vi "Termo_1.5__.vi"() -> ()   [LabVIEW 2015]
doc: "Программа мониторинга температуры и вакуума"
uses:
  tango_vi.llb/avToDoubleScalar.vi
  tango_vi.llb/tango.lvlib
panel:
  out "T1":dbl format="%.2f"
  out "C2":string
  out "C1":string
  out "Т3":dbl format="%.2f"
  out "Т5":dbl format="%.2f"
  out "Т8":dbl format="%.2f"
  out "Т6":dbl format="%.2f"
  out "T14":dbl format="%.2f"
  out "T13":dbl format="%.2f"
  out "Т9":dbl format="%.2f"
  out "Т7":dbl format="%.2f"
  out "PKT2 state":u32(colorbox) caption="ON"
  out "PKT1 state":u32(colorbox) caption="ON"
  out "device name 2":string="kriontube/termo/pkt2"
  out "attribute names 3":string[](array[string])=["R1", "R2", "R3", "R4", "R5", "R6", "R7", "R8"]
  out "Tango device name":string="kriontube/termo/pkt1"
  out "attribute names 2":string[](array[string])=["T1", "T2", "T3", "T4", "T5", "T6", "T7", "T8"]
  out "attribute names":string[](array[string])=["s1_status_byte", "sensor1_P", "sensor2_P", "s2_status_byte"]
  out "Tango device name":string="kriontube/vacuum/tpg361"
  out "Последнее обновление :":string
  out "S 2":string
  out "S 1":string
  out "R13":dbl format="%.2f"
  in  "stop":bool
  out "R9":dbl format="%.2f"
  out "R10":dbl format="%.2f"
  out "R11":dbl format="%.2f"
  out "R12":dbl format="%.2f"
  out "R14":dbl format="%.2f"
  out "R7":dbl format="%.2f"
  out "R5":dbl format="%.2f"
  out "R8":dbl format="%.2f"
  out "R6":dbl format="%.2f"
  out "R3":dbl format="%.2f"
  out "R1":dbl format="%.2f"
  out "R4":dbl format="%.2f"
  out "R2":dbl format="%.2f"
  out "R16":dbl format="%.2f"
  out "R15":dbl format="%.2f"
  out "T12":dbl format="%.2f"
  out "T10":dbl format="%.2f"
  out "T11":dbl format="%.2f"
  out "T4":dbl format="%.2f"
  out "T2":dbl format="%.2f"
  out "TPG 361 state":u32(colorbox) caption="UNKNOWN"
  out "T15":dbl format="%.2f"
  out "T16":dbl format="%.2f"
  # "КРИОН-Т"
  # "4 K"
  # "40 K"
  # "P"
  # "[ mBar ]"
  # "R [Ом]"
  # "R1"
  # "R2"
  # "R3"
  # "R4"
  # "R5"
  # "R6"
  # "R7"
  # "R9"
  # "R8"
  # "R10"
  # "R11"
  # "T1"
  # "R12"
  # "R13"
  # "R14"
  # "Вакуум"
  # "Термометрия \nПКТ8-1 , ПКТ8-2"
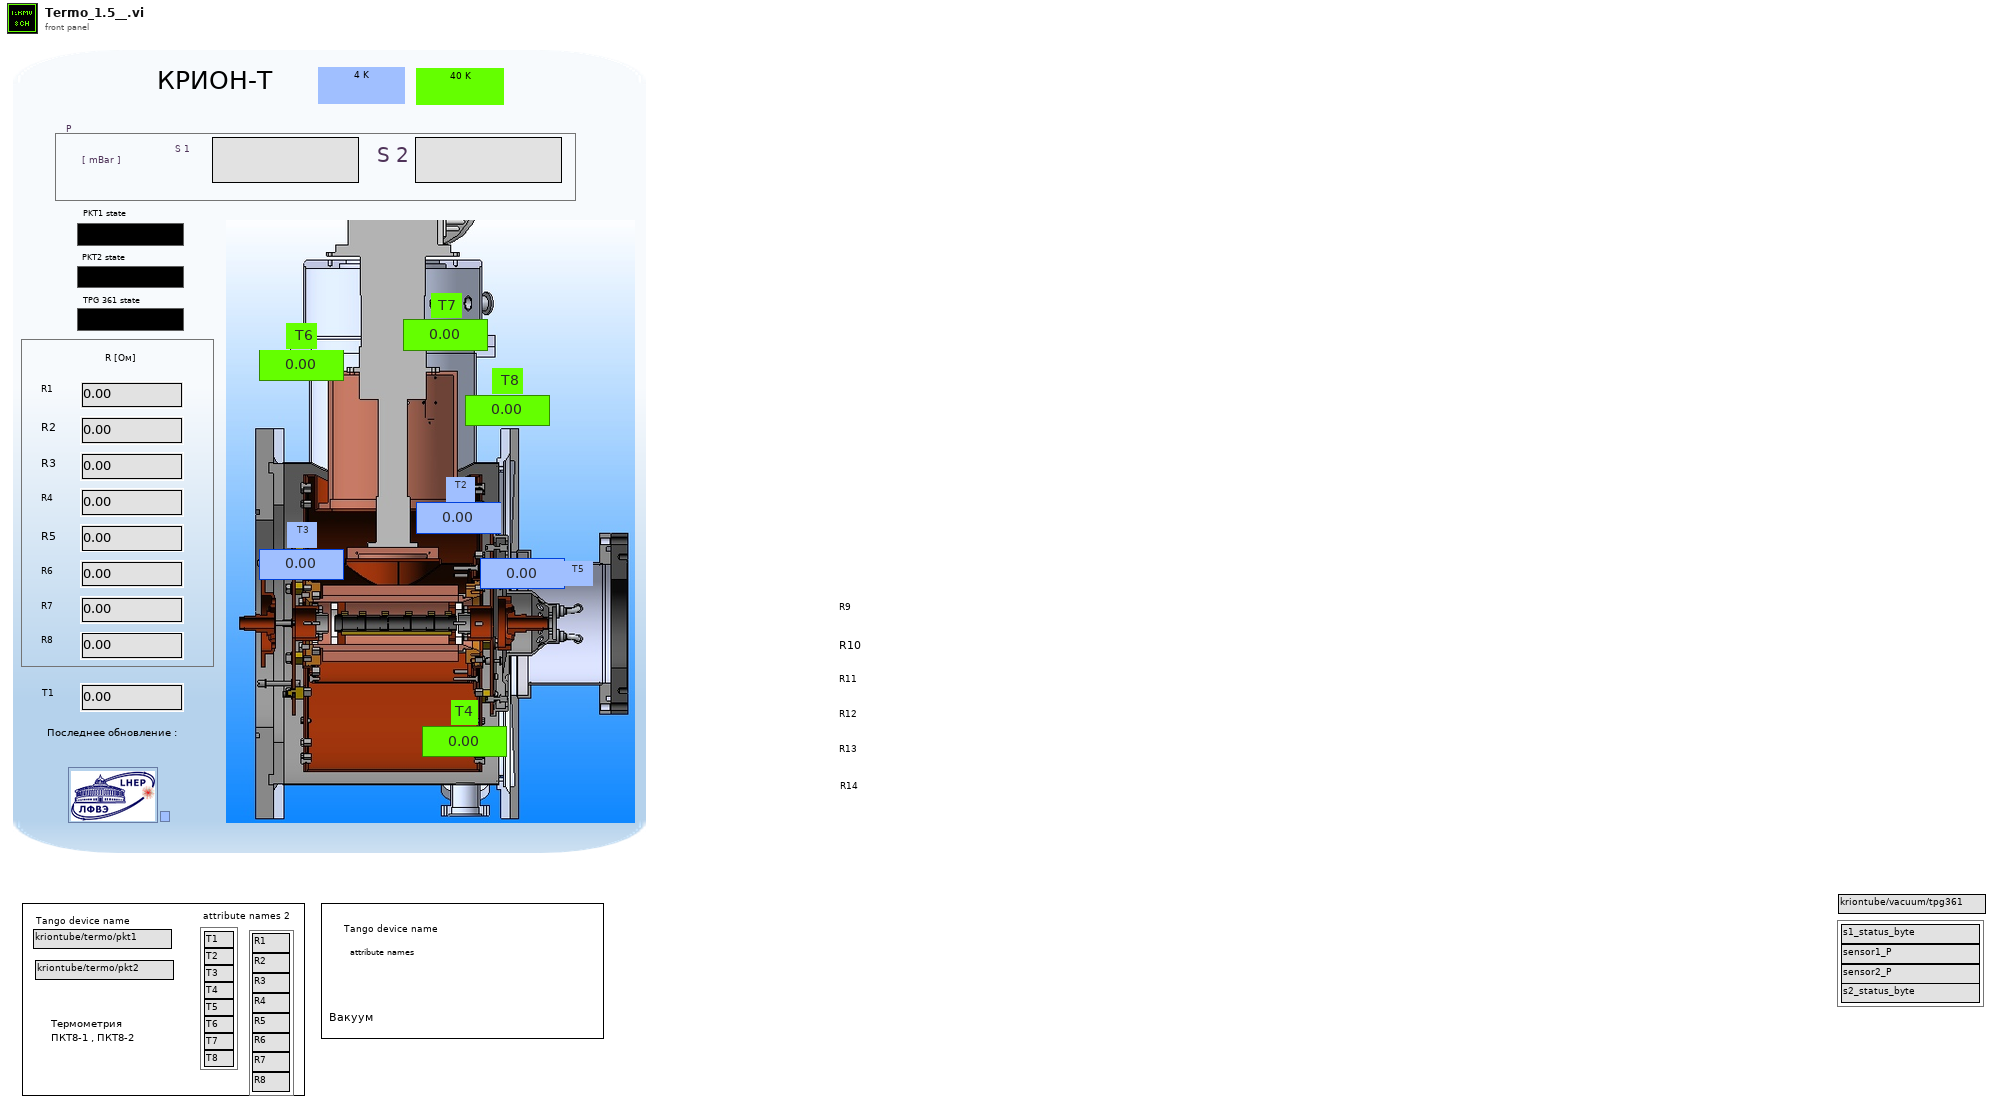
[diagram p1: front panel]
types:
  T1 = cluster{"device name":string, "attribute name":string, "quality value":i16, "quality string":string, "timestamp":dbl, "dim. x":i32, "dim. y":i32, "value":u8[], "error code":i32, "error stack":string[], "data type":u16}[]
  T2 = cluster{"device name":string, "attribute name":string, "quality value":i16, "quality string":string, "timestamp":dbl, "dim. x":i32, "dim. y":i32, "value":u8[], "error code":i32, "error stack":string[], "data type":u16}
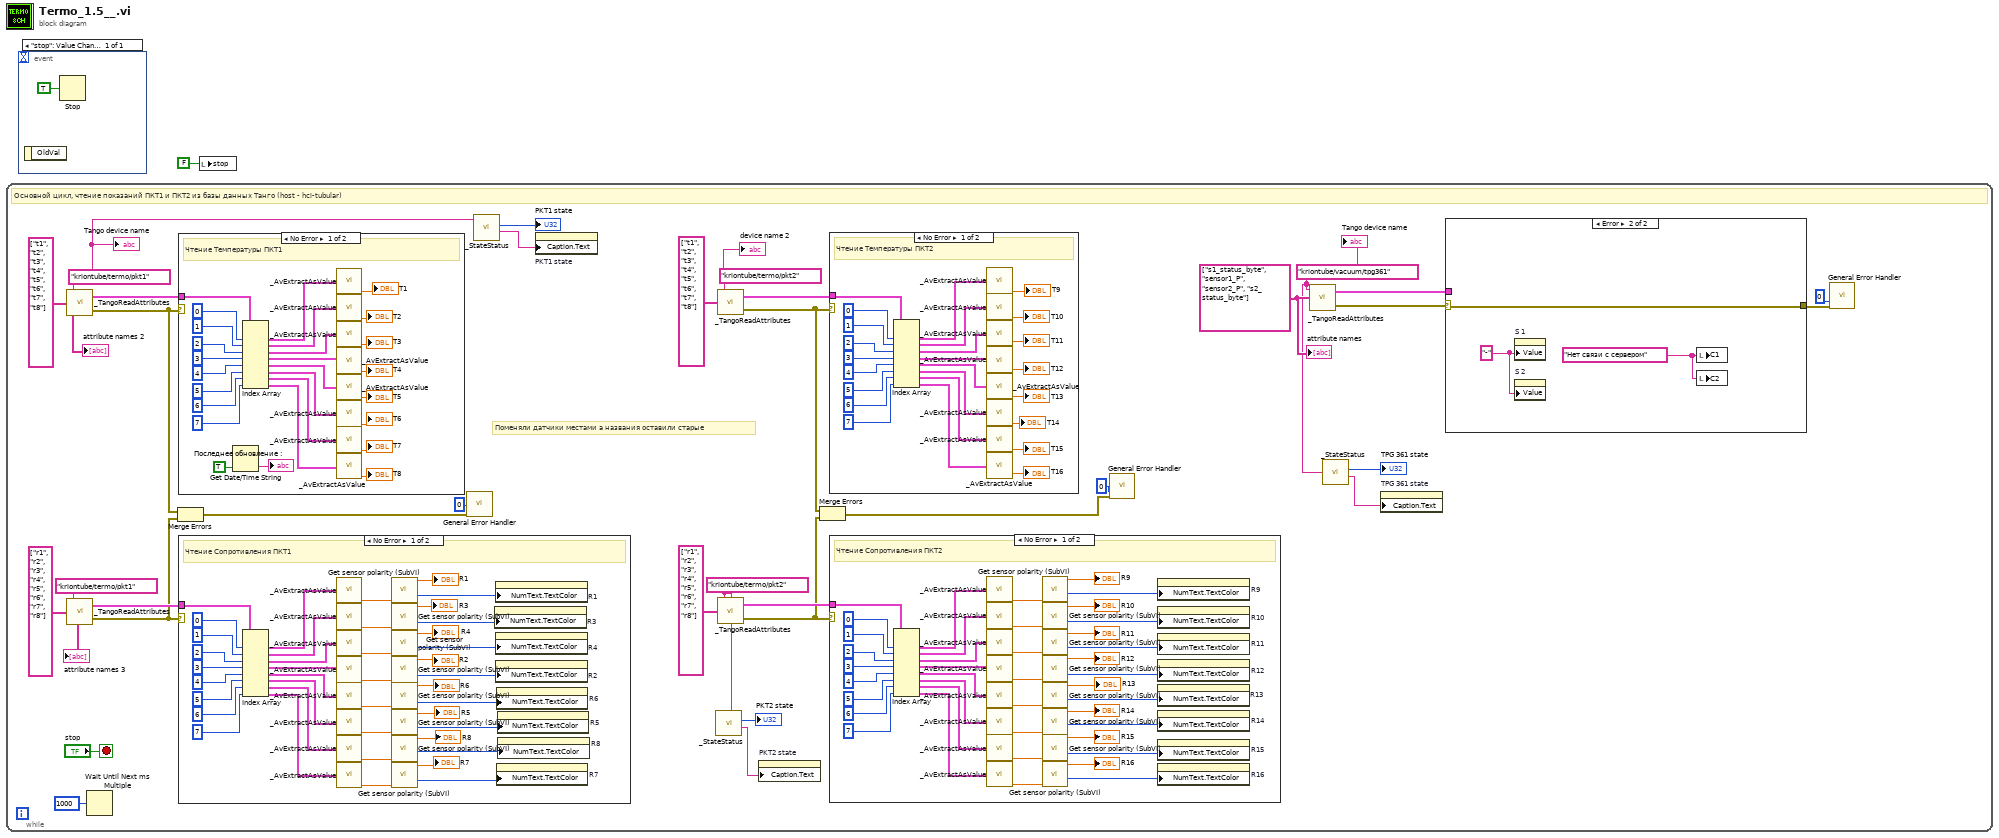
[diagram p0: block diagram]
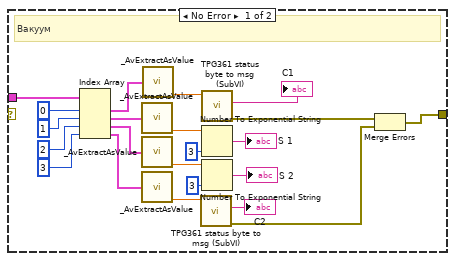
[diagram p2: hidden frame]
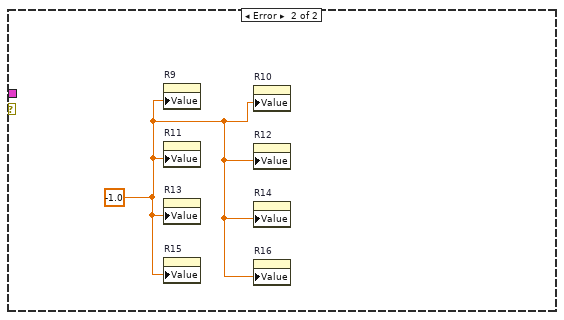
[diagram p3: hidden frame]
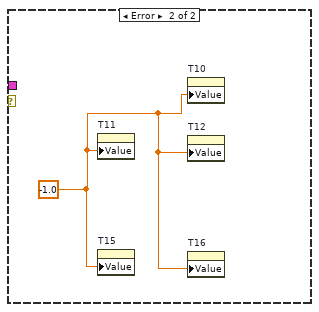
[diagram p4: hidden frame]
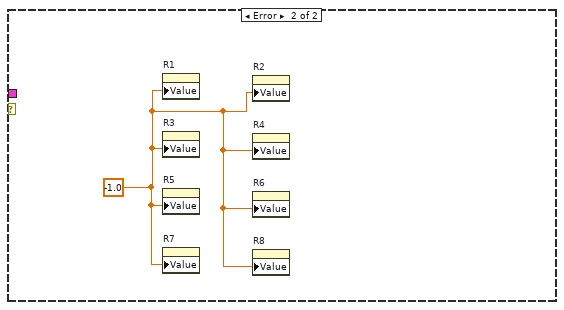
[diagram p5: hidden frame]
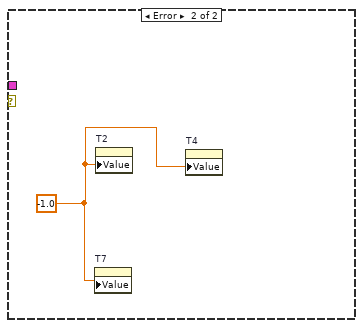
[diagram p6: hidden frame]
diagram:
  n1 = while {
    stop <- "stop" stop-if-true
    w14 = string[] ["s1_status_byte", "sensor1_P", "sensor2_P", "s2_status_byte"] ("attribute names")
    w2 = "kriontube/vacuum/tpg361" ("device name")
    w7 = "kriontube/termo/pkt2" ("device name")
    w26 = "kriontube/termo/pkt2" ("device name")
    w30 = string[] ["r1", "r2", "r3", "r4", "r5", "r6", "r7", "r8"] ("attribute names")
    w11 = "kriontube/termo/pkt1" ("device name")
    w31 = string[] ["t1", "t2", "t3", "t4", "t5", "t6", "t7", "t8"] ("attribute names")
    # "Поменяли датчики местами а названия оставили старые"
    # "Основной цикл, чтение показаний ПКТ1 и ПКТ2 из базы данных Танго (host - hci-tubular)"
    n2 = call "_TangoReadAttributes.vi"("attribute names"=w31, "device name"=w11) -> ("error out"=w23:errorcluster, "attribute values"=w32:T1)  [unwired: 1 in]
    n3 = call "_TangoReadAttributes.vi"("attribute names"=w30, "device name"="kriontube/termo/pkt1") -> ("error out"=w22:errorcluster, "attribute values"=w29:T1)  [unwired: 1 in]
    n4 = Wait Until Next ms Multiple(millisecond multiple=u32 1000) -> ()  [unwired: 1 out]
    n5 = Merge Errors(w23, w22) -> (w21:errorcluster)
    n6 = case shown="No Error" w23 {
      tunnel: w32 -> [w196 _]
      frame No Error {
        # "Чтение Температуры ПКТ1"
        n7 = Get Date/Time String(want seconds? (F)=TRUE) -> (time string=→"Последнее обновление :":string)  [unwired: 2 in, 1 out]
        n8 = Index Array(array=w196, index #1=0 ("indice"), index #2=1 ("index"), index #3=2 ("indice"), index #4=3 ("index"), index #5=4 ("index"), index #6=5 ("indice"), index #7=6 ("index"), index #8=7 ("indice")) -> (element #1=w195:T2, element #2=w190:T2, element #3=w189:T2, element #4=w188:T2, element #5=w187:T2, element #6=w183:T2, element #7=w182:T2, element #8=w181:T2)
        n9 = call-poly "_AvExtractAsValue.vi"("attribute value"=w195) -> ("value"=→"T1":dbl)  [unwired: 4 out]
        n10 = call-poly "_AvExtractAsValue.vi"("attribute value"=w190) -> ("value"=→"T2":dbl)  [unwired: 4 out]
        n11 = call-poly "_AvExtractAsValue.vi"("attribute value"=w189) -> ("value"=→"Т3":dbl)  [unwired: 4 out]
        n12 = call-poly "_AvExtractAsValue.vi"("attribute value"=w188) -> ("value"=→"T4":dbl)  [unwired: 4 out]
        n13 = call-poly "_AvExtractAsValue.vi"("attribute value"=w187) -> ("value"=→"Т5":dbl)  [unwired: 4 out]
        n14 = call-poly "_AvExtractAsValue.vi"("attribute value"=w183) -> ("value"=→"Т6":dbl)  [unwired: 4 out]
        n15 = call-poly "_AvExtractAsValue.vi"("attribute value"=w182) -> ("value"=→"Т7":dbl)  [unwired: 4 out]
        n16 = call-poly "_AvExtractAsValue.vi"("attribute value"=w181) -> ("value"=→"Т8":dbl)  [unwired: 4 out]
      }
      frame Error {
        w198 = -1.0 ("millisecond multiple")
        n17 = property on="Т7" class="DigNum (strict)"("Value"=w198) -> ()  [unwired: 2 in, 2 out]
        n18 = property on="T2" class="DigNum (strict)"("Value"=w198) -> ()  [unwired: 2 in, 2 out]
        n19 = property on="T4" class="DigNum (strict)"("Value"=w198) -> ()  [unwired: 2 in, 2 out]
      }
    }
    n20 = case shown="No Error" w22 {
      tunnel: w29 -> [w168 _]
      frame No Error {
        # "Чтение Сопротивления ПКТ1"
        n21 = Index Array(array=w168, index #1=0 ("indice"), index #2=1 ("index"), index #3=2 ("indice"), index #4=3 ("index"), index #5=4 ("index"), index #6=5 ("indice"), index #7=6 ("index"), index #8=7 ("indice")) -> (element #1=w167:T2, element #2=w162:T2, element #3=w161:T2, element #4=w160:T2, element #5=w159:T2, element #6=w155:T2, element #7=w154:T2, element #8=w153:T2)
        n22 = call-poly "_AvExtractAsValue.vi"("attribute value"=w167) -> ("value"=w152:dbl)  [unwired: 4 out]
        n23 = call-poly "_AvExtractAsValue.vi"("attribute value"=w162) -> ("value"=w151:dbl)  [unwired: 4 out]
        n24 = call-poly "_AvExtractAsValue.vi"("attribute value"=w161) -> ("value"=w150:dbl)  [unwired: 4 out]
        n25 = call-poly "_AvExtractAsValue.vi"("attribute value"=w160) -> ("value"=w149:dbl)  [unwired: 4 out]
        n26 = call-poly "_AvExtractAsValue.vi"("attribute value"=w159) -> ("value"=w148:dbl)  [unwired: 4 out]
        n27 = call-poly "_AvExtractAsValue.vi"("attribute value"=w155) -> ("value"=w147:dbl)  [unwired: 4 out]
        n28 = call-poly "_AvExtractAsValue.vi"("attribute value"=w154) -> ("value"=w146:dbl)  [unwired: 4 out]
        n29 = call-poly "_AvExtractAsValue.vi"("attribute value"=w153) -> ("value"=w145:dbl)  [unwired: 4 out]
        n30 = call "Get sensor polarity (SubVI).vi"("R вх"=w152) -> ("R по модулю"=→"R1":dbl, "Цвет полярности вкл. R"=w143:u32)  [unwired: 13 in]
        n31 = call "Get sensor polarity (SubVI).vi"("R вх"=w151) -> ("R по модулю"=→"R3":dbl, "Цвет полярности вкл. R"=w141:u32)  [unwired: 13 in]
        n32 = call "Get sensor polarity (SubVI).vi"("R вх"=w150) -> ("R по модулю"=→"R4":dbl, "Цвет полярности вкл. R"=w139:u32)  [unwired: 13 in]
        n33 = call "Get sensor polarity (SubVI).vi"("R вх"=w149) -> ("R по модулю"=→"R2":dbl, "Цвет полярности вкл. R"=w137:u32)  [unwired: 13 in]
        n34 = call "Get sensor polarity (SubVI).vi"("R вх"=w148) -> ("R по модулю"=→"R6":dbl, "Цвет полярности вкл. R"=w135:u32)  [unwired: 13 in]
        n35 = call "Get sensor polarity (SubVI).vi"("R вх"=w147) -> ("R по модулю"=→"R5":dbl, "Цвет полярности вкл. R"=w133:u32)  [unwired: 13 in]
        n36 = call "Get sensor polarity (SubVI).vi"("R вх"=w146) -> ("R по модулю"=→"R8":dbl, "Цвет полярности вкл. R"=w131:u32)  [unwired: 13 in]
        n37 = call "Get sensor polarity (SubVI).vi"("R вх"=w145) -> ("R по модулю"=→"R7":dbl, "Цвет полярности вкл. R"=w129:u32)  [unwired: 13 in]
        n38 = property on="R3" class="DigNum (strict)"("NumText.TextColor"=w141) -> ()  [unwired: 2 in, 2 out]
        n39 = property on="R1" class="DigNum (strict)"("NumText.TextColor"=w143) -> ()  [unwired: 2 in, 2 out]
        n40 = property on="R4" class="DigNum (strict)"("NumText.TextColor"=w139) -> ()  [unwired: 2 in, 2 out]
        n41 = property on="R2" class="DigNum (strict)"("NumText.TextColor"=w137) -> ()  [unwired: 2 in, 2 out]
        n42 = property on="R6" class="DigNum (strict)"("NumText.TextColor"=w135) -> ()  [unwired: 2 in, 2 out]
        n43 = property on="R7" class="DigNum (strict)"("NumText.TextColor"=w129) -> ()  [unwired: 2 in, 2 out]
        n44 = property on="R5" class="DigNum (strict)"("NumText.TextColor"=w133) -> ()  [unwired: 2 in, 2 out]
        n45 = property on="R8" class="DigNum (strict)"("NumText.TextColor"=w131) -> ()  [unwired: 2 in, 2 out]
      }
      frame Error {
        w170 = -1.0 ("millisecond multiple")
        n46 = property on="R1" class="DigNum (strict)"("Value"=w170) -> ()  [unwired: 2 in, 2 out]
        n47 = property on="R3" class="DigNum (strict)"("Value"=w170) -> ()  [unwired: 2 in, 2 out]
        n48 = property on="R5" class="DigNum (strict)"("Value"=w170) -> ()  [unwired: 2 in, 2 out]
        n49 = property on="R7" class="DigNum (strict)"("Value"=w170) -> ()  [unwired: 2 in, 2 out]
        n50 = property on="R2" class="DigNum (strict)"("Value"=w170) -> ()  [unwired: 2 in, 2 out]
        n51 = property on="R4" class="DigNum (strict)"("Value"=w170) -> ()  [unwired: 2 in, 2 out]
        n52 = property on="R6" class="DigNum (strict)"("Value"=w170) -> ()  [unwired: 2 in, 2 out]
        n53 = property on="R8" class="DigNum (strict)"("Value"=w170) -> ()  [unwired: 2 in, 2 out]
      }
    }
    n54 = call <vilib>:"General Error Handler.vi"("type of dialog (OK msg:1)"=u32 0 ("milliseconds to wait"), "error in (no error)"=w21) -> ()  [unwired: 1 in, 13 out]
    n55 = call "_StateStatus.vi"("Device Name"=w11) -> ("State Color"=→"PKT1 state":u32, "State String"=w6:string)  [unwired: 4 out]
    n56 = property on="PKT1 state" class="ColBox"("Caption.Text"=w6) -> ()  [unwired: 2 in, 2 out]
    n57 = call "_StateStatus.vi"("Device Name"=w7) -> ("State Color"=→"PKT2 state":u32, "State String"=w5:string)  [unwired: 4 out]
    n58 = call "_TangoReadAttributes.vi"("attribute names"=string[] ["t1", "t2", "t3", "t4", "t5", "t6", "t7", "t8"], "device name"=w26) -> ("error out"=w19:errorcluster, "attribute values"=w24:T1)  [unwired: 1 in]
    n59 = call "_TangoReadAttributes.vi"("attribute names"=string[] ["r1", "r2", "r3", "r4", "r5", "r6", "r7", "r8"], "device name"=w7) -> ("error out"=w18:errorcluster, "attribute values"=w28:T1)  [unwired: 1 in]
    n60 = property on="PKT2 state" class="ColBox"("Caption.Text"=w5) -> ()  [unwired: 2 in, 2 out]
    n61 = Merge Errors(w19, w18) -> (w17:errorcluster)
    n62 = case shown="No Error" w19 {
      tunnel: w24 -> [w126 _]
      frame No Error {
        # "Чтение Температуры ПКТ2"
        n63 = Index Array(array=w126, index #1=0 ("indice"), index #2=1 ("index"), index #3=2 ("indice"), index #4=3 ("index"), index #5=4 ("index"), index #6=5 ("indice"), index #7=6 ("index"), index #8=7 ("indice")) -> (element #1=w125:T2, element #2=w120:T2, element #3=w119:T2, element #4=w118:T2, element #5=w117:T2, element #6=w113:T2, element #7=w112:T2, element #8=w111:T2)
        n64 = call-poly "_AvExtractAsValue.vi"("attribute value"=w125) -> ("value"=→"Т9":dbl)  [unwired: 4 out]
        n65 = call-poly "_AvExtractAsValue.vi"("attribute value"=w120) -> ("value"=→"T10":dbl)  [unwired: 4 out]
        n66 = call-poly "_AvExtractAsValue.vi"("attribute value"=w119) -> ("value"=→"T11":dbl)  [unwired: 4 out]
        n67 = call-poly "_AvExtractAsValue.vi"("attribute value"=w118) -> ("value"=→"T12":dbl)  [unwired: 4 out]
        n68 = call-poly "_AvExtractAsValue.vi"("attribute value"=w117) -> ("value"=→"T13":dbl)  [unwired: 4 out]
        n69 = call-poly "_AvExtractAsValue.vi"("attribute value"=w113) -> ("value"=→"T14":dbl)  [unwired: 4 out]
        n70 = call-poly "_AvExtractAsValue.vi"("attribute value"=w112) -> ("value"=→"T15":dbl)  [unwired: 4 out]
        n71 = call-poly "_AvExtractAsValue.vi"("attribute value"=w111) -> ("value"=→"T16":dbl)  [unwired: 4 out]
      }
      frame Error {
        w128 = -1.0 ("millisecond multiple")
        n72 = property on="T11" class="DigNum (strict)"("Value"=w128) -> ()  [unwired: 2 in, 2 out]
        n73 = property on="T15" class="DigNum (strict)"("Value"=w128) -> ()  [unwired: 2 in, 2 out]
        n74 = property on="T10" class="DigNum (strict)"("Value"=w128) -> ()  [unwired: 2 in, 2 out]
        n75 = property on="T12" class="DigNum (strict)"("Value"=w128) -> ()  [unwired: 2 in, 2 out]
        n76 = property on="T16" class="DigNum (strict)"("Value"=w128) -> ()  [unwired: 2 in, 2 out]
      }
    }
    n77 = case shown="No Error" w18 {
      tunnel: w28 -> [w100 _]
      frame No Error {
        # "Чтение Сопротивления ПКТ2"
        n78 = Index Array(array=w100, index #1=0 ("indice"), index #2=1 ("index"), index #3=2 ("indice"), index #4=3 ("index"), index #5=4 ("index"), index #6=5 ("indice"), index #7=6 ("index"), index #8=7 ("indice")) -> (element #1=w99:T2, element #2=w94:T2, element #3=w93:T2, element #4=w92:T2, element #5=w91:T2, element #6=w87:T2, element #7=w86:T2, element #8=w85:T2)
        n79 = call-poly "_AvExtractAsValue.vi"("attribute value"=w99) -> ("value"=w84:dbl)  [unwired: 4 out]
        n80 = call-poly "_AvExtractAsValue.vi"("attribute value"=w94) -> ("value"=w83:dbl)  [unwired: 4 out]
        n81 = call-poly "_AvExtractAsValue.vi"("attribute value"=w93) -> ("value"=w82:dbl)  [unwired: 4 out]
        n82 = call-poly "_AvExtractAsValue.vi"("attribute value"=w92) -> ("value"=w81:dbl)  [unwired: 4 out]
        n83 = call-poly "_AvExtractAsValue.vi"("attribute value"=w91) -> ("value"=w63:dbl)  [unwired: 4 out]
        n84 = call-poly "_AvExtractAsValue.vi"("attribute value"=w87) -> ("value"=w80:dbl)  [unwired: 4 out]
        n85 = call-poly "_AvExtractAsValue.vi"("attribute value"=w86) -> ("value"=w79:dbl)  [unwired: 4 out]
        n86 = call-poly "_AvExtractAsValue.vi"("attribute value"=w85) -> ("value"=w78:dbl)  [unwired: 4 out]
        n87 = call "Get sensor polarity (SubVI).vi"("R вх"=w84) -> ("R по модулю"=→"R9":dbl, "Цвет полярности вкл. R"=w70:u32)  [unwired: 13 in]
        n88 = call "Get sensor polarity (SubVI).vi"("R вх"=w83) -> ("R по модулю"=→"R10":dbl, "Цвет полярности вкл. R"=w69:u32)  [unwired: 13 in]
        n89 = call "Get sensor polarity (SubVI).vi"("R вх"=w82) -> ("R по модулю"=→"R11":dbl, "Цвет полярности вкл. R"=w68:u32)  [unwired: 13 in]
        n90 = call "Get sensor polarity (SubVI).vi"("R вх"=w81) -> ("R по модулю"=→"R12":dbl, "Цвет полярности вкл. R"=w67:u32)  [unwired: 13 in]
        n91 = call "Get sensor polarity (SubVI).vi"("R вх"=w63) -> ("R по модулю"=→"R13":dbl, "Цвет полярности вкл. R"=w61:u32)  [unwired: 13 in]
        n92 = call "Get sensor polarity (SubVI).vi"("R вх"=w80) -> ("R по модулю"=→"R14":dbl, "Цвет полярности вкл. R"=w66:u32)  [unwired: 13 in]
        n93 = call "Get sensor polarity (SubVI).vi"("R вх"=w79) -> ("R по модулю"=→"R15":dbl, "Цвет полярности вкл. R"=w65:u32)  [unwired: 13 in]
        n94 = call "Get sensor polarity (SubVI).vi"("R вх"=w78) -> ("R по модулю"=→"R16":dbl, "Цвет полярности вкл. R"=w64:u32)  [unwired: 13 in]
        n95 = property on="R9" class="DigNum (strict)"("NumText.TextColor"=w70) -> ()  [unwired: 2 in, 2 out]
        n96 = property on="R10" class="DigNum (strict)"("NumText.TextColor"=w69) -> ()  [unwired: 2 in, 2 out]
        n97 = property on="R11" class="DigNum (strict)"("NumText.TextColor"=w68) -> ()  [unwired: 2 in, 2 out]
        n98 = property on="R12" class="DigNum (strict)"("NumText.TextColor"=w67) -> ()  [unwired: 2 in, 2 out]
        n99 = property on="R13" class="DigNum (strict)"("NumText.TextColor"=w61) -> ()  [unwired: 2 in, 2 out]
        n100 = property on="R14" class="DigNum (strict)"("NumText.TextColor"=w66) -> ()  [unwired: 2 in, 2 out]
        n101 = property on="R15" class="DigNum (strict)"("NumText.TextColor"=w65) -> ()  [unwired: 2 in, 2 out]
        n102 = property on="R16" class="DigNum (strict)"("NumText.TextColor"=w64) -> ()  [unwired: 2 in, 2 out]
      }
      frame Error {
        w102 = -1.0 ("millisecond multiple")
        n103 = property on="R9" class="DigNum (strict)"("Value"=w102) -> ()  [unwired: 2 in, 2 out]
        n104 = property on="R11" class="DigNum (strict)"("Value"=w102) -> ()  [unwired: 2 in, 2 out]
        n105 = property on="R13" class="DigNum (strict)"("Value"=w102) -> ()  [unwired: 2 in, 2 out]
        n106 = property on="R15" class="DigNum (strict)"("Value"=w102) -> ()  [unwired: 2 in, 2 out]
        n107 = property on="R10" class="DigNum (strict)"("Value"=w102) -> ()  [unwired: 2 in, 2 out]
        n108 = property on="R12" class="DigNum (strict)"("Value"=w102) -> ()  [unwired: 2 in, 2 out]
        n109 = property on="R14" class="DigNum (strict)"("Value"=w102) -> ()  [unwired: 2 in, 2 out]
        n110 = property on="R16" class="DigNum (strict)"("Value"=w102) -> ()  [unwired: 2 in, 2 out]
      }
    }
    n111 = call <vilib>:"General Error Handler.vi"("type of dialog (OK msg:1)"=u32 0 ("milliseconds to wait"), "error in (no error)"=w17) -> ()  [unwired: 1 in, 13 out]
    n112 = call "_TangoReadAttributes.vi"("attribute names"=w14, "device name"=w2) -> ("error out"=w15:errorcluster, "attribute values"=w16:T1)  [unwired: 1 in]
    n113 = call "_StateStatus.vi"("Device Name"=w2) -> ("State Color"=→"TPG 361 state":u32, "State String"=w3:string)  [unwired: 4 out]
    n114 = property on="TPG 361 state" class="ColBox"("Caption.Text"=w3) -> ()  [unwired: 2 in, 2 out]
    n115 = case shown="Error" w15 {
      selector: w15 -> [_ w59]
      tunnel: w16 -> [w57 _]
      tunnel: [w38 w59] -> w12
      frame No Error {
        # "Вакуум"
        n116 = Index Array(array=w57, index #1=0 ("indice"), index #2=1 ("index"), index #3=2 ("indice"), index #4=3 ("index")) -> (element #1=w44:T2, element #2=w49:T2, element #3=w45:T2, element #4=w42:T2)
        n117 = call-poly "_AvExtractAsValue.vi"("attribute value"=w49) -> ("value"=w52:dbl)  [unwired: 4 out]
        n118 = call-poly "_AvExtractAsValue.vi"("attribute value"=w45) -> ("value"=w47:dbl)  [unwired: 4 out]
        n119 = call-poly "_AvExtractAsValue.vi"("attribute value"=w42) -> ("value"=w41:dbl)  [unwired: 4 out]
        n120 = call-poly "_AvExtractAsValue.vi"("attribute value"=w44) -> ("value"=w43:dbl)  [unwired: 4 out]
        n121 = call "TPG361 status byte to msg (SubVI).vi"("In Error number"=w41) -> ("error out"=w39:errorcluster, "Статус сообщение"=→"C2":string)  [unwired: 9 in]
        n122 = call "TPG361 status byte to msg (SubVI).vi"("In Error number"=w43) -> ("error out"=w40:errorcluster, "Статус сообщение"=→"C1":string)  [unwired: 9 in]
        n123 = Number To Exponential String(number=w52, precision (6)=i16 3) -> (E-format string=→"S 1":string)  [unwired: 2 in]
        n124 = Number To Exponential String(number=w47, precision (6)=i16 3) -> (E-format string=→"S 2":string)  [unwired: 2 in]
        n125 = Merge Errors(w40, w39) -> (w38:errorcluster)
      }
      frame Error {
        w58 = "Нет связи с сервером" ("PrdStatus")
        w60 = "-" ("Sensor 1")
        n126 = property on="S 1" class="Str"("Value"=w60) -> ()  [unwired: 2 in, 2 out]
        n127 = property on="S 2" class="Str"("Value"=w60) -> ()  [unwired: 2 in, 2 out]
        n128 = local write "C1"(w58) -> ()
        n129 = local write "C2"(w58) -> ()
      }
    }
    n130 = call <vilib>:"General Error Handler.vi"("type of dialog (OK msg:1)"=u32 0 ("milliseconds to wait"), "error in (no error)"=w12) -> ()  [unwired: 1 in, 13 out]
    "Tango device name" <- w2
    "attribute names" <- w14
    "attribute names 2" <- w31
    "Tango device name" <- w11
    "attribute names 3" <- w30
    "device name 2" <- w26
  }
  n131 = event shown="[0] \"stop\": Value Change" {
    selector: _ -> [_]
    dyn-events: _ -> [_]
    timeout: _ -> [_]
    event "stop": Value Change {
      n132 = event-data() -> ()  [unwired: 1 in, 1 out]
      n133 = Stop(stop? (T)=TRUE) -> ()
    }
  }
  n134 = local write "stop"(FALSE ("Boolean")) -> ()
